vi "tipshaping.vi"(8 "error in (no error)":errorcluster, 11 "Input":string="34,45,89") -> (0 "error out":errorcluster, 3 "Output":string)   [LabVIEW 2014]
uses:
  <userlib>/Nanonis Prog Interface V5/Nanonis Prog Interface.lvlib
panel:
  in  "milliseconds to wait":u32
  out "size(s)":i32=3
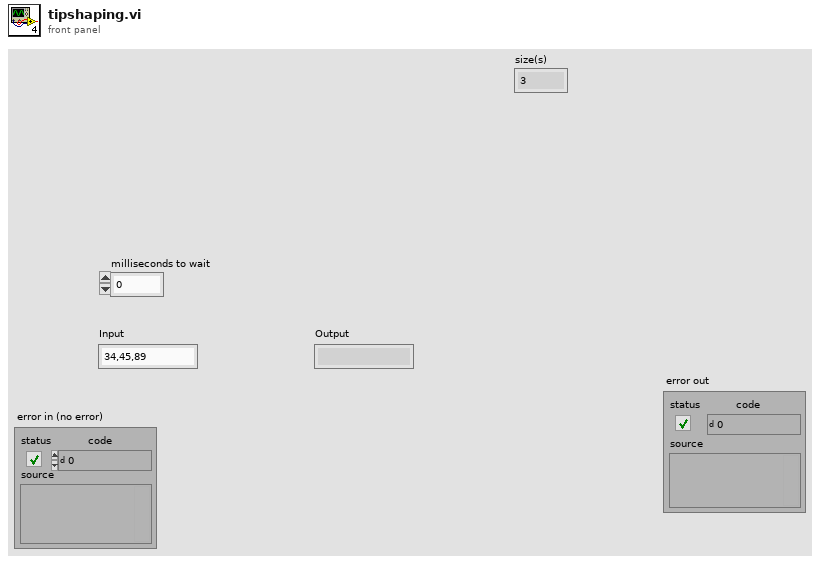
[diagram p1: front panel]
types:
  T1 = cluster{"TipLift":dbl, "Bias Settling Time":dbl, "Lift Height":dbl, "Lift Time 2":dbl, "Lifting Bias":dbl, "Lift Time 1":dbl}
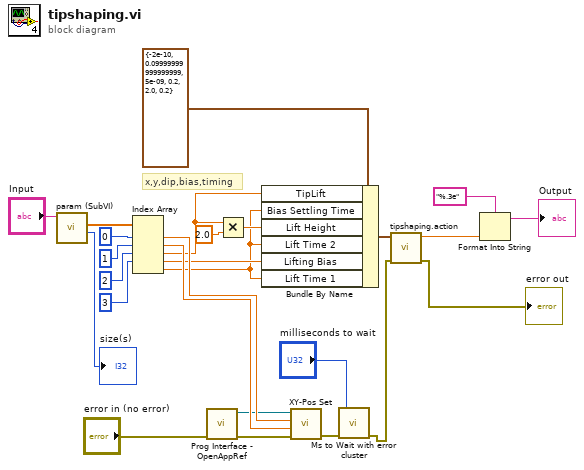
[diagram p0: block diagram]
diagram:
  # "x,y,dip,bias,timing"
  n1 = call <userlib>:"param (SubVI).vi"("Input"="Input") -> ("num"=→"size(s)":i32, "parm"=w24:dbl[])  [unwired: 8 in, 1 out]
  n2 = Index Array(array=w24, index #1=0 ("index"), index #2=1 ("index"), index #3=2 ("index"), index #4=3 ("index")) -> (element #1=w13:dbl, element #2=w12:dbl, element #3=w8:dbl, element #4=w5:dbl, element #5=w4:dbl)  [unwired: 1 in]
  n3 = call <userlib>:"Prog Interface - OpenAppRef.vi"("Error in (no error)"="error in (no error)") -> ("Error out"=w10:errorcluster, "Application reference"=w11:refnum<vi>)  [unwired: 5 in]
  n4 = Multiply(x=w8, y=2.0) -> (x*y=w7:dbl)
  n5 = Bundle By Name(cluster=T1 {"TipLift"=-2e-10, "Bias Settling Time"=0.09999999999999999, "Lift Height"=5e-09, "Lift Time 2"=0.2, "Lifting Bias"=2.0, "Lift Time 1"=0.2} ("TipShapingParam"), "TipLift"=w8, "Bias Settling Time"=w4, "Lift Height"=w7, "Lift Time 2"=w4, "Lifting Bias"=w5, "Lift Time 1"=w4) -> (w14:T1)
  n6 = call <userlib>:"XY-Pos Set.vi"("error in (no error)"=w10, "Y (m)"=w12, "X (m)"=w13, "Application ref in"=w11) -> ("error out"=w2:errorcluster)  [unwired: 4 in, 1 out]
  n7 = call <userlib>:"Ms to Wait with error cluster.vi"("error in (no error)"=w2, "milliseconds to wait"="milliseconds to wait") -> ("error out"=w3:errorcluster)  [unwired: 4 in, 1 out]
  n8 = call <userlib>:"tipshaping.action.vi"("Error in (no error)"=w3, "TipShapingParam"=w14) -> ("error out"=→"error out":errorcluster, "dz"=w17:sgl)  [unwired: 8 in]
  n9 = Format Into String(format string="%.3e", w17) -> (resulting string=→"Output":string)  [unwired: 2 in, 1 out]
